vi "Pure Pursuit_New (Sub VI).vi"(0 "x_lat_path":dbl[](array[numeric]), 2 "L":dbl format="%#_13g", 5 "y_long_path":dbl[](array[numeric]), 7 "X_Current":dbl format="%#_13g", 9 "Y_Current":dbl format="%#_13g", 11 "Heading_Current":dbl format="%#_13g", 12 "#pnt":i32, 13 "WP no_pre":i32, 14 "LAD":dbl format="%#_13g") -> (4 "Steer_CMD(Deg)":dbl, 15 "Index(near vehicle)":i32)   [LabVIEW 2020]
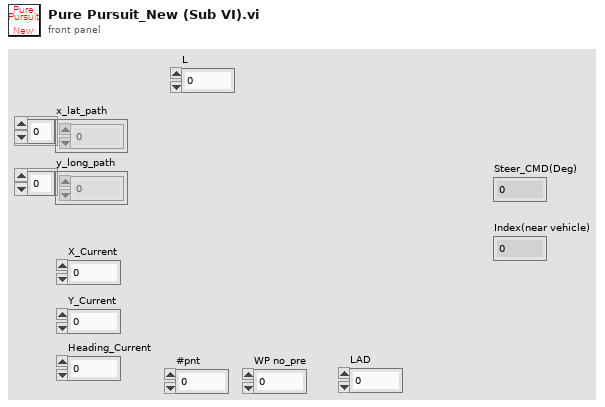
[diagram p1: front panel]
types:
  T1 = cluster{"Dist. WP":dbl, "Index":i32, "Heading_lane":dbl, "Dist. lane":dbl}
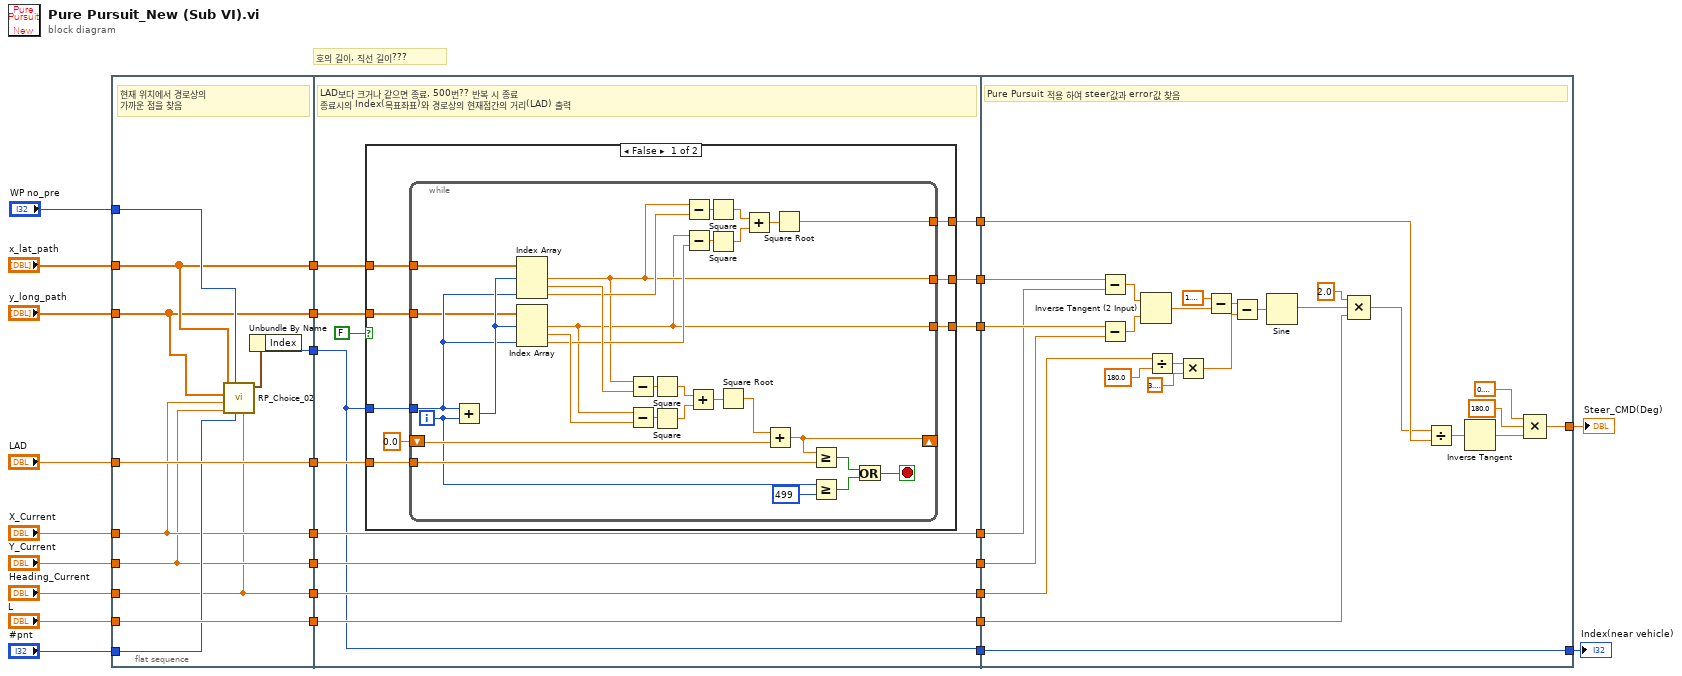
[diagram p0: block diagram]
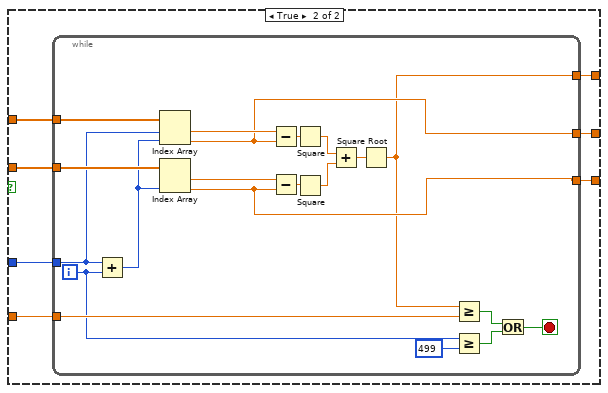
[diagram p2: hidden frame]
diagram:
  # "호의 길이, 직선 길이???"
  n1 = flat-sequence {
    tunnel: "x_lat_path" -> [w34]
    tunnel: [w34] -> w27
    tunnel: "y_long_path" -> [w33]
    tunnel: [w33] -> w25
    tunnel: "LAD" -> [w38]
    tunnel: [w38] -> w22
    tunnel: "X_Current" -> [w32]
    tunnel: "Y_Current" -> [w31]
    tunnel: [w32] -> w16
    tunnel: [w31] -> w15
    tunnel: "Heading_Current" -> [w28]
    tunnel: [w28] -> w11
    tunnel: "L" -> [w37]
    tunnel: [w37] -> w7
    tunnel: "WP no_pre" -> [w36]
    tunnel: "#pnt" -> [w35]
    tunnel: [w29] -> w1
    tunnel: w27 -> [w50]
    tunnel: w25 -> [w49]
    tunnel: w22 -> [w48]
    tunnel: [w47] -> w21
    tunnel: [w46] -> w20
    tunnel: [w45] -> w19
    tunnel: w16 -> [w44]
    tunnel: w15 -> [w43]
    tunnel: [w44] -> w14
    tunnel: [w43] -> w13
    tunnel: w11 -> [w42]
    tunnel: [w42] -> w10
    tunnel: [w41] -> w9
    tunnel: w7 -> [w41]
    tunnel: [w39] -> w6
    tunnel: w1 -> [w39]
    tunnel: w21 -> [w135]
    tunnel: w20 -> [w130]
    tunnel: w19 -> [w129]
    tunnel: w14 -> [w127]
    tunnel: w13 -> [w126]
    tunnel: w10 -> [w121]
    tunnel: w9 -> [w117]
    tunnel: w6 -> [w141]
    tunnel: [w141] -> w5
    tunnel: [w137] -> w4
    frame #0 {
      # "현재 위치에서 경로상의\n가까운 점을 찾음"
      n2 = call "RP_Choice_02.vi"("Heading_c"=w28, "# of pnt"=w35, "WP no_pre"=w36, "y_long_c"=w31, "x_lat_c"=w32, "y_long_arr"=w33, "x_lat_arr"=w34) -> ("RP1"=w30:T1)  [unwired: 1 in, 3 out]
      n3 = Unbundle By Name(w30) -> ("Index"=w29:i32)
    }
    frame #1 {
      # "LAD보다 크거나 같으면 종료, 500번?? 반복 시 종료\n종료시의 Index(목표좌표)와 경로상의 현재점간의 거리(LAD) 출력"
      n4 = case shown="False" FALSE {
        tunnel: w39 -> [w55 w95]
        tunnel: w50 -> [w57 w94]
        tunnel: w49 -> [w56 w93]
        tunnel: w48 -> [w51 w92]
        tunnel: [w52 w91] -> w47
        tunnel: [w53 w90] -> w46
        tunnel: [w54 w89] -> w45
        frame False {
          n5 = while {
            tunnel: w55 -> [w87]
            tunnel: w57 -> [w81]
            tunnel: w56 -> [w80]
            tunnel: w51 -> [w75]
            shift-right: [w74] -> _
            shift-left: 0.0 -> [w76]
            tunnel: [w61] -> w52
            tunnel: [w60] -> w53
            tunnel: [w59] -> w54
            i -> [w70]
            stop <- w71 stop-if-true
            n6 = Add(x=w87, y=w70) -> (x+y=w88:i32)
            n7 = Index Array(array=w81, index #1=w88, index #3=w87) -> (element #1=w60:dbl, element #2=w79:dbl, element #3=w63:dbl)  [unwired: 1 in]
            n8 = Index Array(array=w80, index #1=w88, index #3=w87) -> (element #1=w59:dbl, element #2=w78:dbl, element #3=w62:dbl)  [unwired: 1 in]
            n9 = Subtract(x=w60, y=w79) -> (x-y=w85:dbl)
            n10 = Subtract(x=w59, y=w78) -> (x-y=w86:dbl)
            n11 = Square(x=w85) -> (x^2=w84:dbl)
            n12 = Square(x=w86) -> (x^2=w83:dbl)
            n13 = Subtract(x=w60, y=w63) -> (x-y=w65:dbl)
            n14 = Subtract(x=w59, y=w62) -> (x-y=w64:dbl)
            n15 = Add(x=w84, y=w83) -> (x+y=w82:dbl)
            n16 = Square(x=w65) -> (x^2=w66:dbl)
            n17 = Square(x=w64) -> (x^2=w67:dbl)
            n18 = Square Root(x=w82) -> (sqrt(x)=w77:dbl)
            n19 = Add(x=w66, y=w67) -> (x+y=w68:dbl)
            n20 = Add(x=w77, y=w76) -> (x+y=w74:dbl)
            n21 = Square Root(x=w68) -> (sqrt(x)=w61:dbl)
            n22 = Greater Or Equal?(x=w74, y=w75) -> (x >= y?=w73:bool)
            n23 = Greater Or Equal?(x=w70, y=499) -> (x >= y?=w72:bool)
            n24 = Or(x=w73, y=w72) -> (x .or. y?=w71:bool)
          }
        }
        frame True {
          n25 = while {
            tunnel: w95 -> [w101]
            tunnel: w94 -> [w110]
            tunnel: w93 -> [w109]
            tunnel: w92 -> [w108]
            tunnel: [w96] -> w91
            tunnel: [w98] -> w90
            tunnel: [w97] -> w89
            i -> [w104]
            stop <- w105 stop-if-true
            n26 = Add(x=w101, y=w104) -> (x+y=w102:i32)
            n27 = Index Array(array=w110, index #1=w101, index #2=w102) -> (element #1=w100:dbl, element #2=w98:dbl)
            n28 = Index Array(array=w109, index #2=w102) -> (element #1=w99:dbl, element #2=w97:dbl)  [unwired: 1 in]
            n29 = Subtract(x=w100, y=w98) -> (x-y=w114:dbl)
            n30 = Subtract(x=w99, y=w97) -> (x-y=w115:dbl)
            n31 = Square(x=w114) -> (x^2=w113:dbl)
            n32 = Square(x=w115) -> (x^2=w112:dbl)
            n33 = Add(x=w113, y=w112) -> (x+y=w111:dbl)
            n34 = Square Root(x=w111) -> (sqrt(x)=w96:dbl)
            n35 = Greater Or Equal?(x=w96, y=w108) -> (x >= y?=w107:bool)
            n36 = Greater Or Equal?(x=w104, y=499) -> (x >= y?=w106:bool)
            n37 = Or(x=w107, y=w106) -> (x .or. y?=w105:bool)
          }
        }
      }
    }
    frame #2 {
      # "Pure Pursuit 적용 하여 steer값과 error값 찾음"
      n38 = Subtract(x=w130, y=w127) -> (x-y=w134:dbl)
      n39 = Subtract(x=w129, y=w126) -> (x-y=w133:dbl)
      n40 = Inverse Tangent (2 Input)(1:w133, 2:w134) -> (0:w132:dbl)
      n41 = Divide(x=w121, y=180.0) -> (x/y=w125:dbl)
      n42 = Multiply(x=w125, y=3.141592653589793) -> (x*y=w123:dbl)
      n43 = Subtract(x=1.5707963267948966, y=w132) -> (x-y=w131:dbl)
      n44 = Subtract(x=w131, y=w123) -> (x-y=w120:dbl)
      n45 = Sine(x=w120) -> (sin(x)=w118:dbl)
      n46 = Compound Arithmetic op=MULTIPLY(2.0, w118, w117) -> (w116:dbl)
      n47 = Divide(x=w116, y=w135) -> (x/y=w136:dbl)
      n48 = Inverse Tangent(1:w136) -> (0:w138:dbl)
      n49 = Compound Arithmetic op=MULTIPLY(0.3183098861837907, 180.0, w138) -> (w137:dbl)
    }
  }
  "Steer_CMD(Deg)" <- w4
  "Index(near vehicle)" <- w5
